vi "Add New Feature.vi"(8 "error in":errorcluster) -> (0 "error out":errorcluster, 2 "New Feature":string, 3 "Add New?":bool)   [LabVIEW 2024]
uses:
  Buttons/Cancel.ctl
panel:
  in  "New Feature Name:":string
  in  "OK Button":bool
  in  "Cancel Button":T1
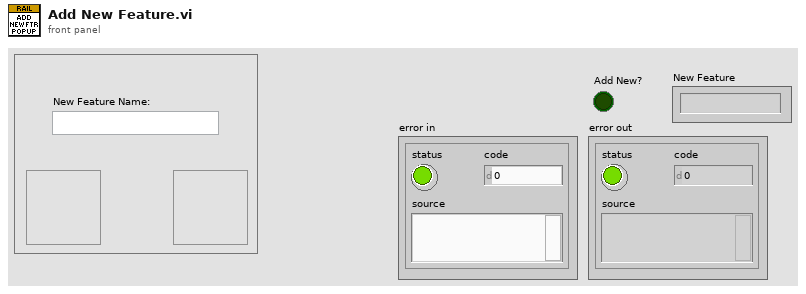
[diagram p1: front panel]
types:
  T1 = typedef "Cancel.ctl" = bool
  T2 = enum8{"Enabled", "Disabled", "Disabled and Grayed Out"}
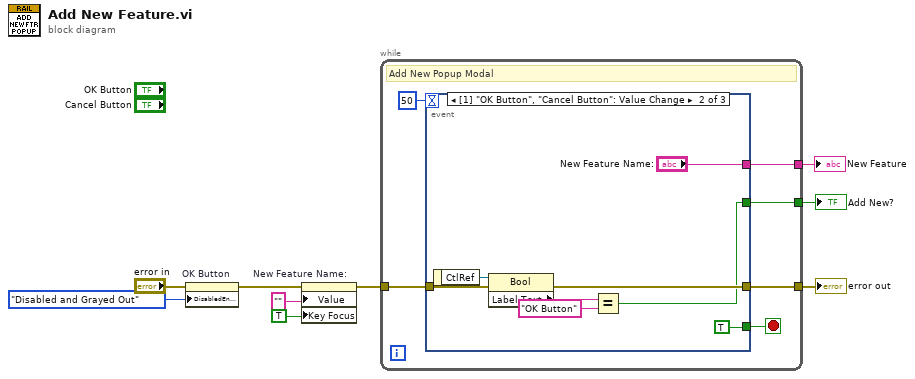
[diagram p0: block diagram]
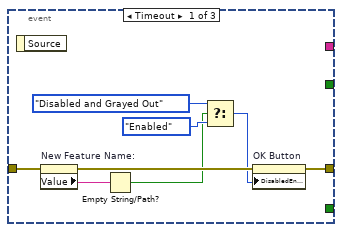
[diagram p2: hidden frame]
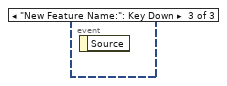
[diagram p3: hidden frame]
diagram:
  n1 = property on="OK Button" class="Bool"(error in="error in", "DisabledEnum"=T2."Disabled and Grayed Out" ("Disabled")) -> (error out=w4:errorcluster)  [unwired: 1 in, 1 out]
  n2 = property on="New Feature Name:" class="Str"(error in=w4, "Value"="" ("New Feature Name:"), "Key Focus"=TRUE) -> (error out=w3:errorcluster)  [unwired: 1 in, 1 out]
  n3 = while {
    tunnel: w3 -> [w14]
    tunnel: [w13] -> w9
    tunnel: [w11] -> w6
    tunnel: [w10] -> w5
    stop <- w12 stop-if-true
    # "Add New Popup Modal"
    n4 = event shown="[1] \"OK Button\", \"Cancel Button\": Value Change" {
      selector: _ -> [_ _ _]
      dyn-events: _ -> [_ _ _]
      timeout: 50 -> [_ _ _]
      tunnel: w14 -> [w23 w31 _]
      tunnel: [w20 w28 _] -> w13
      tunnel: [_ TRUE _] -> w12
      tunnel: [_ w24 _] -> w11
      tunnel: [_ "New Feature Name:" _] -> w10
      event Timeout {
        n5 = event-data() -> ()  [unwired: 1 in, 1 out]
        n6 = property on="New Feature Name:" class="Str"(error in=w23) -> (error out=w21:errorcluster, "Value"=w22:string)  [unwired: 1 in, 1 out]
        n7 = Empty String/Path?(string/path=w22) -> (empty?=w17:bool)
        n8 = Select(t=T2."Disabled and Grayed Out" ("Disabled"), s=w17, f=T2."Enabled" ("Disabled")) -> (s? t:f=w16:T2)
        n9 = property on="OK Button" class="Bool"(error in=w21, "DisabledEnum"=w16) -> (error out=w20:errorcluster)  [unwired: 1 in, 1 out]
      }
      event "OK Button": Value Change {
        n10 = event-data() -> ("CtlRef"=w27:refnum<vi>)  [unwired: 1 in]
        n11 = property class="Bool"(reference=w27, error in=w31) -> (error out=w28:errorcluster, "Label.Text"=w26:string)  [unwired: 1 out]
        n12 = Equal?(x=w26, y="OK Button") -> (x = y?=w24:bool)
      }
      event "New Feature Name:": Key Down {
        n13 = event-data() -> ()  [unwired: 1 in, 1 out]
      }
    }
  }
  "error out" <- w9
  "Add New?" <- w6
  "New Feature" <- w5
